vi "x-direction.vi"(4 "keypressed [4]":dbl, 5 "keypressed [2]":dbl, 6 "keypressed [3]":dbl, 7 "keypressed [1]":dbl, 8 "keypressed [0]":dbl, 10 "xback":dbl, 11 "xfwd":dbl) -> (2 "xback":bool, 3 "xfwd":bool)   [LabVIEW 2011]
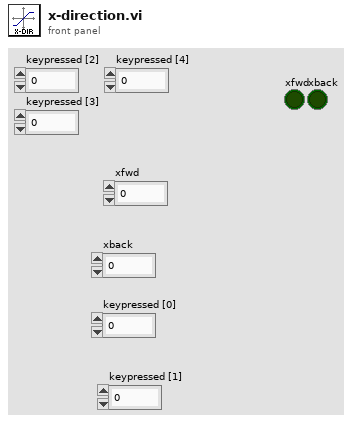
[diagram p1: front panel]
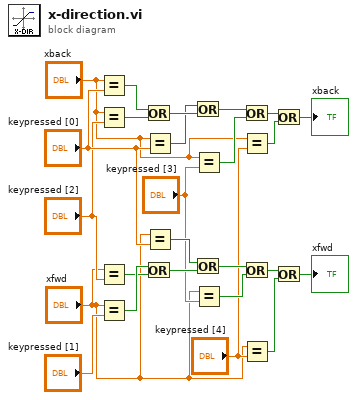
[diagram p0: block diagram]
diagram:
  n1 = Equal?(x="xback", y="keypressed [0]") -> (x = y?=w16:bool)
  n2 = Equal?(x="xback", y="keypressed [2]") -> (x = y?=w15:bool)
  n3 = Equal?(x="xfwd", y="keypressed [2]") -> (x = y?=w18:bool)
  n4 = Equal?(x="xfwd", y="keypressed [1]") -> (x = y?=w19:bool)
  n5 = Or(x=w16, y=w15) -> (x .or. y?=w24:bool)
  n6 = Or(x=w19, y=w18) -> (x .or. y?=w25:bool)
  n7 = Equal?(x="xback", y="keypressed [0]") -> (x = y?=w17:bool)
  n8 = Equal?(x="xfwd", y="keypressed [0]") -> (x = y?=w20:bool)
  n9 = Or(x=w17, y=w24) -> (x .or. y?=w13:bool)
  n10 = Or(x=w20, y=w25) -> (x .or. y?=w10:bool)
  n11 = Equal?(x="xback", y="keypressed [3]") -> (x = y?=w12:bool)
  n12 = Equal?(x="xfwd", y="keypressed [3]") -> (x = y?=w11:bool)
  n13 = Or(x=w13, y=w12) -> (x .or. y?=w6:bool)
  n14 = Equal?(x="xback", y="keypressed [4]") -> (x = y?=w7:bool)
  n15 = Or(x=w10, y=w11) -> (x .or. y?=w5:bool)
  n16 = Equal?(x="xfwd", y="keypressed [4]") -> (x = y?=w4:bool)
  n17 = Or(x=w6, y=w7) -> (x .or. y?=→"xback":bool)
  n18 = Or(x=w5, y=w4) -> (x .or. y?=→"xfwd":bool)
